vi "fringe_creation.vi"(7 "flip fringe direction":bool, 8 "fringe number":u32, 9 "phase shift":dbl(knob) min=0.0 max=6.28 scale=0.0..6.28, 10 "yPixel":i32, 11 "xPixel":i32) -> (2 "Image":T1(plugin-control))   [LabVIEW 2011]
panel:
  in  "Boolean":bool
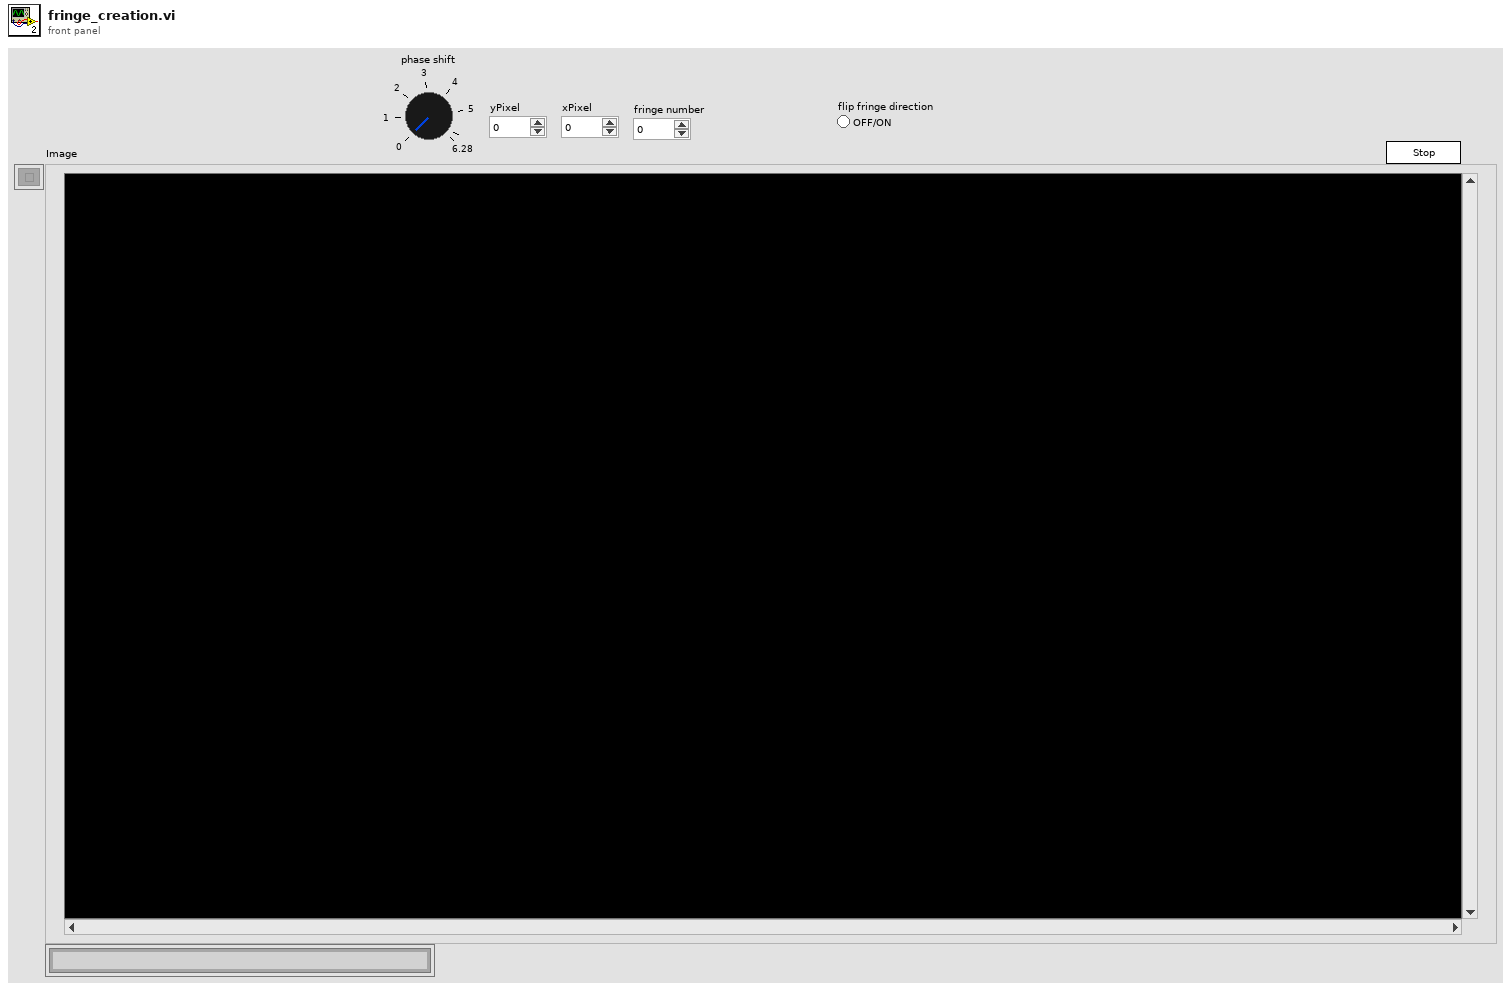
[diagram p1: front panel]
types:
  T1 = typedef "IMAQ Image.ctl" = refnum<image>
  T2 = typedef "Image Type" = u32
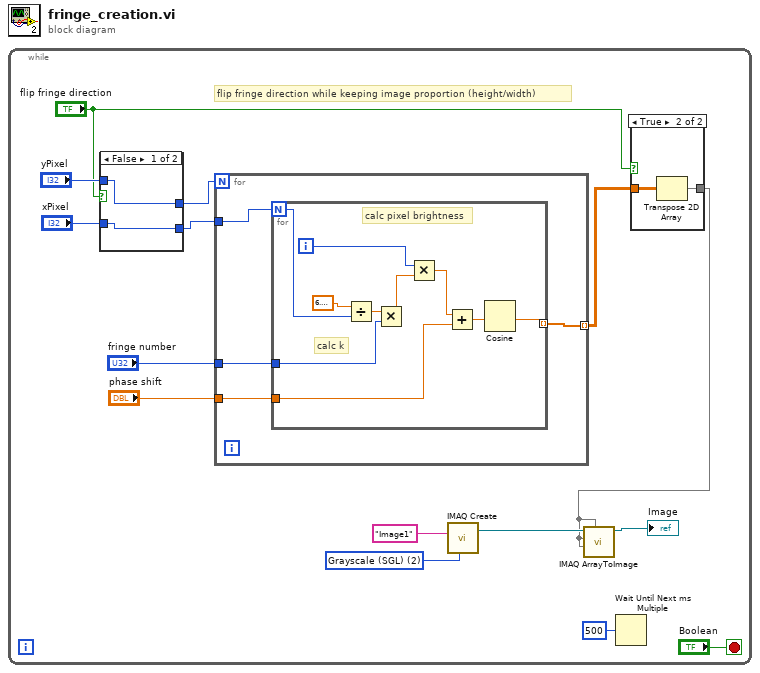
[diagram p0: block diagram]
diagram:
  n1 = while {
    stop <- "Boolean" stop-if-true
    w8 = T2 2 items=["Grayscale (U8)", "Grayscale (I16)", "Grayscale (SGL)", "Complex (CSG)", "RGB (U32)", "HSL (U32)", "RGB (U64)", "Grayscale (U16)"] ("Image Type")
    # "flip fringe direction while keeping image proportion (height/width)"
    n2 = case shown="False" "flip fringe direction" {
      tunnel: "yPixel" -> [w17 w19]
      tunnel: "xPixel" -> [w16 w18]
      tunnel: [w16 w19] -> w5
      tunnel: [w17 w18] -> w4
      frame False {
      }
      frame True {
      }
    }
    n3 = for {
      N: w4 -> [_]
      tunnel: [w26] -> w10 mode=indexing
      tunnel: w5 -> [w25]
      tunnel: "fringe number" -> [w24]
      tunnel: "phase shift" -> [w23]
      n4 = for {
        N: w25 -> [w34]
        tunnel: [w31] -> w26 mode=indexing
        tunnel: w24 -> [w30]
        tunnel: w23 -> [w28]
        i -> [w35]
        # "calc pixel brightness"
        # "calc k"
        n5 = Divide(x=6.283185307179586, y=w34) -> (x/y=w33:dbl)
        n6 = Multiply(x=w33, y=w30) -> (x*y=w32:dbl)
        n7 = Multiply(x=w35, y=w32) -> (x*y=w29:dbl)
        n8 = Add(x=w29, y=w28) -> (x+y=w27:dbl)
        n9 = Cosine(x=w27) -> (cos(x)=w31:dbl)
      }
    }
    n10 = call "IMAQ Create"("Image Name"="Image1", "Image Type"=w8) -> ("New Image"=w14:T1)  [unwired: 2 in, 2 out]
    n11 = Wait Until Next ms Multiple(millisecond multiple=u32 500) -> ()  [unwired: 1 out]
    n12 = case shown="True" "flip fringe direction" {
      tunnel: w10 -> [w20 w22]
      tunnel: [w20 w21] -> w9
      frame False {
      }
      frame True {
        n13 = Transpose 2D Array(2D array=w22) -> (transposed array=w21:dbl[][])
      }
    }
    n14 = call "IMAQ ArrayToImage"("Image Pixels (Float)"=w9, "Image Pixels (U16)"=w9, "Image Pixels (I16)"=w9, "Image Pixels (U8)"=w9, "Image"=w14) -> ("Image Out"=→"Image":T1)  [unwired: 5 in, 1 out]
  }
